vi "IsHotGoalCRIO.vi"(8 "error in":errorcluster, 9 "% Cutoff":dbl, 10 "Num samples":i32) -> (0 "error out":errorcluster, 2 "Hot/Not":bool)   [LabVIEW 2013]
doc: "IsHotGoalCRIO checks if the goal is hot at the beginning of autonomous mode. Image processing is done on the CRIO.\n-NumSamples determines how many images of the goal the camera will process.\n-% Cutoff (meant to be a decimal value) determines the minimum ratio of hot images/total images needed for IsHotGoal to report a hot goal. For example, if .6 was the % cutoff, then at least 60% of images would need to be hot."
uses:
  Example_Code/2014 Target Detection/TargetType.ctl
panel:
  out "Iterations":i32
  in  "Color System":u16(ring)=2 items=["RGB", "HSL", "HSV", "HSI"]
  in  "Score cutoff":dbl=50.0
  out "Distance (ft)":dbl
  out "Scores.State":T1
  in  "Color Components":T2={"Hue"={116.0, 148.0}, "Sat"={152.0, 255.0}, "Val"={237.0, 255.0}} {"Val" scale=0.0..255.0; "Sat" scale=0.0..255.0; "Hue" scale=0.0..255.0 scale format="%#_3g"}
  out "Time (ms)":u32
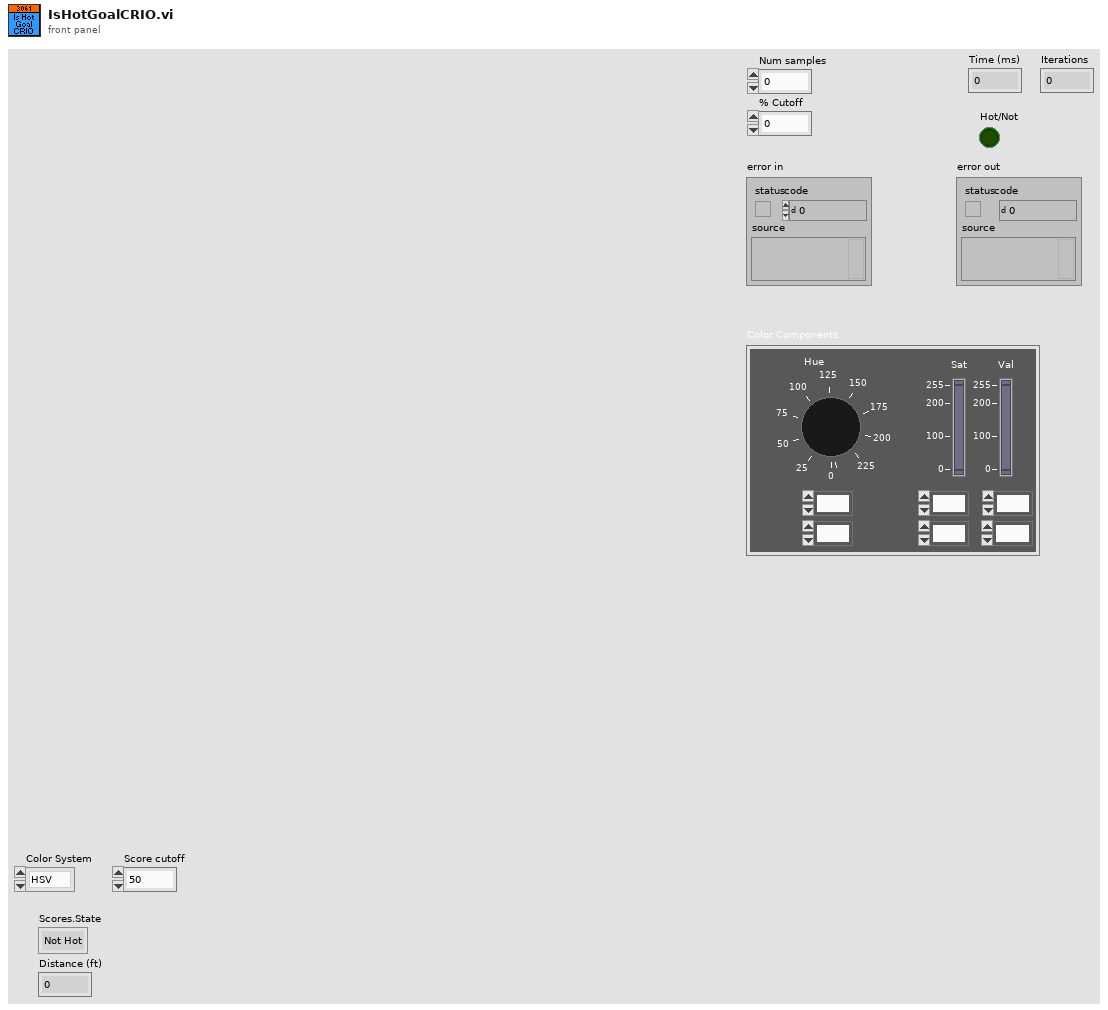
[diagram p1: front panel]
types:
  T1 = typedef "TargetType.ctl" = enum16{"Not Hot", "Hot"}
  T2 = cluster{"Hue":cluster{dbl, dbl}, "Sat":cluster{dbl, dbl}, "Val":cluster{dbl, dbl}}
  T3 = typedef "Image Type" = u32
  T4 = typedef "WPI_CameraDevRef.ctl" = cluster{"Camera Address":string, "CameraStatus":errorcluster, "Acquire Image Notifier":refnum<notifier>}
  T5 = typedef "IMAQ Image.ctl" = refnum<image>
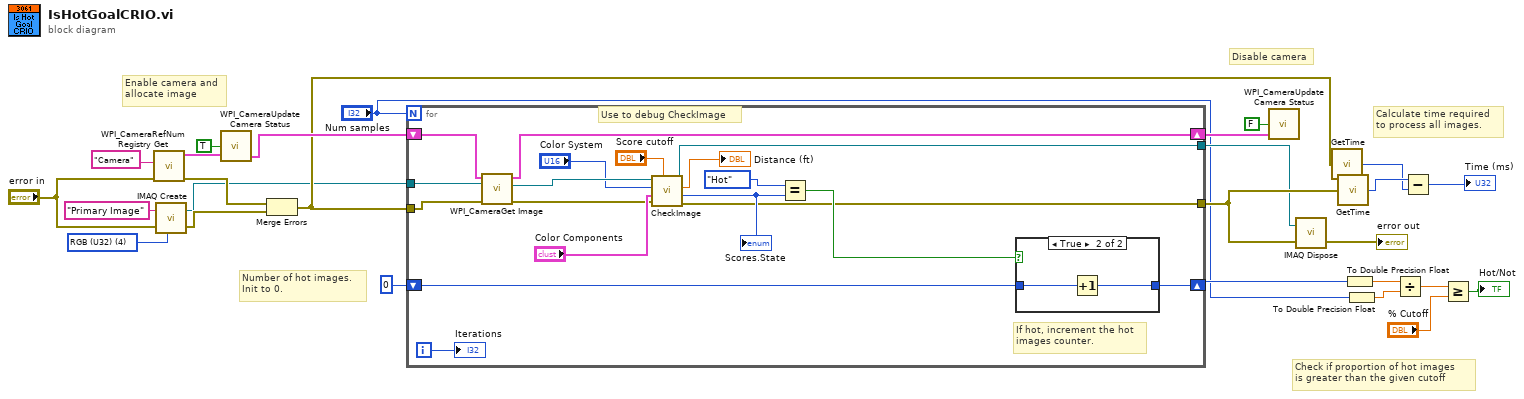
[diagram p0: block diagram]
diagram:
  w15 = T3 4 items=["Grayscale (U8)", "Grayscale (I16)", "Grayscale (SGL)", "Complex (CSG)", "RGB (U32)", "HSL (U32)", "RGB (U64)"] ("Image Type")
  # "Disable camera"
  # "Enable camera and\nallocate image"
  # "Calculate time required \nto process all images."
  # "Check if proportion of hot images\nis greater than the given cutoff"
  # "Number of hot images.\nInit to 0."
  n1 = call <vilib>:"WPI_CameraRefNum Registry Get.vi"("error in (no error)"="error in", "refnum name"="Camera") -> ("error out"=w11:errorcluster, "CameraDevRef"=w18:T4)  [unwired: 8 in]
  n2 = call "IMAQ Create"("Image Name"="Primary Image", "Image Type"=w15, "error in (no error)"="error in") -> ("New Image"=w9:T5, "error out"=w12:errorcluster)  [unwired: 1 in, 1 out]
  n3 = call <vilib>:"WPI_CameraUpdate Camera Status.vi"("CameraDevRef In"=w18, "Enable Vision"=TRUE) -> ("CameraDevRef Out"=w16:T4)  [unwired: 3 in]
  n4 = Merge Errors(w11, w12) -> (w10:errorcluster)
  n5 = for {
    N: "Num samples" -> [_]
    tunnel: w10 -> [w34]
    shift-right: [w44] -> w23
    shift-left: 0 ("Num samples 2") -> [w45]
    tunnel: [w31] -> w6
    tunnel: w9 -> [w35]
    shift-right: [w30] -> w8
    shift-left: w16 -> [w33]
    tunnel: [w29] -> w4
    i -> [w28]
    # "Use to debug CheckImage"
    # "If hot, increment the hot\nimages counter."
    n6 = call <vilib>:"WPI_CameraGet Image.vi"("error in (no error)"=w34, "Image"=w35, "CameraDevRef"=w33) -> ("error out"=w32:errorcluster, "Image Out"=w43:T5, "CameraDevRef Out"=w30:T4)  [unwired: 6 out]
    n7 = call "CheckImage.vi"("Score cutoff"="Score cutoff", "error in"=w32, "Color Components"="Color Components", "Color System"="Color System", "Image"=w43) -> ("error out"=w31:errorcluster, "Scores.State"=w37:T1, "Distance (ft)"=→"Distance (ft)":dbl, "Image out"=w29:T5)  [unwired: 3 in]
    "Scores.State" <- w37
    n8 = Equal?(x=TargetType."Hot" ("Scores.State 2"), y=w37) -> (x = y?=w36:bool)
    n9 = case shown="True" w36 {
      tunnel: w45 -> [w46 w48]
      tunnel: [w46 w47] -> w44
      frame False {
      }
      frame True {
        n10 = Increment(x=w48) -> (x+1=w47:i32)
      }
    }
    "Iterations" <- w28
  }
  n11 = call <vilib>:"WPI_CameraUpdate Camera Status.vi"("CameraDevRef In"=w8, "Enable Vision"=FALSE) -> ()  [unwired: 3 in, 1 out]
  n12 = call "IMAQ Dispose"("Image"=w4, "error in (no error)"=w6) -> ("error out"=→"error out":errorcluster)  [unwired: 4 in]
  n13 = call "GetTime.vi"("error in"=w10) -> ("Time"=w2:u32)
  n14 = call "GetTime.vi"("error in"=w6) -> ("Time"=w3:u32)
  n15 = To Double Precision Float(number=w23) -> (double precision float=w21:dbl)
  n16 = To Double Precision Float(number="Num samples") -> (double precision float=w22:dbl)
  n17 = Divide(x=w21, y=w22) -> (x/y=w24:dbl)
  n18 = Subtract(x=w3, y=w2) -> (x-y=→"Time (ms)":u32)
  n19 = Greater Or Equal?(x=w24, y="% Cutoff") -> (x >= y?=→"Hot/Not":bool)
